vi "Menu Create.vi"(2 "error in":errorcluster, 3 "String":string, 4 "menubar in":refnum<k9>) -> (0 "error out":errorcluster, 1 "menubar out":refnum<k9>)   [LabVIEW 2011]
doc: "<b>通过字符串生成菜单</b>\n<b>格式</b>： Level:M1<T+F+A+m1>,M2<F+T+B+m2>,...,Mn<F+T+N+mn>;\n上述格式为一个菜单分句的示例，上述示例表示向菜单Level中插入M1到Mn共n项子菜单，菜单项M后的括号内的“<b>T+F+A+m1</b>”定义菜单的快捷键和项名称，此部分可以省略。\n\n快捷键定义为<b>Ctrl+Shift+Key</b>，<b>T</b>=<b>包括该按键</b>，<b>F</b>=<b>不包括该按键</b>，后面的<b>m1<mn></b>用于定义菜单项名称，为空则菜单项名称与菜单标识符名称相当。\n<b>Level</b>=<b>Top</b>时，表示向顶级菜单中插入。\n\n注：1.菜单句之间须用<b>:</b>分隔，菜单句中不能出现回车，换行等白字符；\n 2.<b>[分隔符]</b> 用于向菜单插入分隔符"
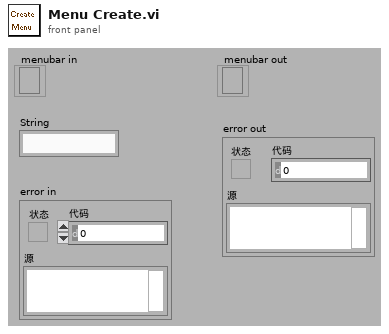
[diagram p1: front panel]
types:
  T1 = typedef "LVMenuShortCut.ctl" = cluster{"Include Shift Key?":bool, "Include Ctrl Key?":bool, "Shortcut Key":string}
  T2 = cluster{"项标识符":string, "项名称":string, "快捷方式":T1}[]
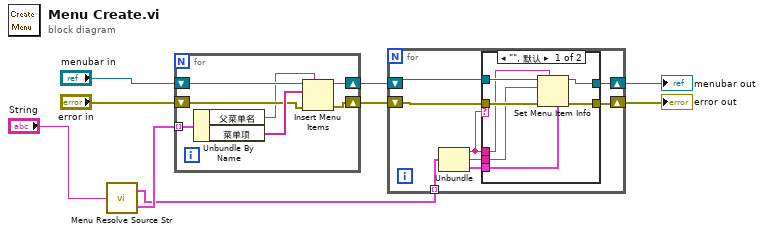
[diagram p0: block diagram]
diagram:
  n1 = call "Menu Resolve Source Str.vi"("字符串"="String") -> ("菜单信息"=w6:cluster{"父菜单名":string, "菜单项":string[]}[], "菜单详情"=w3:T2)
  n2 = for {
    tunnel: w6 -> [w16] mode=indexing
    shift-right: [w13] -> w5
    shift-left: "menubar in" -> [w14]
    shift-right: [w11] -> w4
    shift-left: "error in" -> [w12]
    n3 = Unbundle By Name(w16) -> ("父菜单名"=w10:string, "菜单项"=w15:string[])
    n4 = Insert Menu Items(5:w10, 6:w12, 8:w15, 9:w14) -> (0:w11:errorcluster, 3:w13:refnum<k9>)  [unwired: 3 out]
  }
  n5 = for {
    shift-right: [w18] -> w1
    shift-left: w4 -> [w23]
    shift-right: [w19] -> w2
    shift-left: w5 -> [w24]
    tunnel: w3 -> [w22] mode=indexing
    n6 = Unbundle(w22) -> ("项标识符"=w17:string, "项名称"=w21:string, "快捷方式"=w20:T1)
    n7 = case shown="\"\", 默认" w17 {
      tunnel: w24 -> [w31 w33]
      tunnel: w23 -> [w30 w32]
      tunnel: w17 -> [w29 _]
      tunnel: w21 -> [w28 _]
      tunnel: w20 -> [w27 _]
      tunnel: [w26 w33] -> w19
      tunnel: [w25 w32] -> w18
      frame "", Default {
        n8 = Set Menu Item Info(4:w27, 7:w29, 8:w30, 10:w28, 11:w31) -> (0:w25:errorcluster, 3:w26:refnum<k9>)  [unwired: 2 in]
      }
      frame "APP_SEPARATOR" {
      }
    }
  }
  "error out" <- w1
  "menubar out" <- w2
